vi "BK9120 Main Panel.vi"() -> ()   [LabVIEW 2014]
uses:
  BK9120/Serial_Config.ctl
  Meter_VI.ctl
  BK9120/B&K Precision 9120 series.lvclass
  <vilib>/Utility/error.llb/DialogType.ctl
panel:
  out "Const. Current":bool
  out "Const. Voltage":bool
  out "Enabled":bool
  in  "Output Enable":bool
  in  "Limit Setpoint":T1={"Voltage"=1.0, "Current"=1.0} caption="Measured" {"Current" min=0.0 max=1.2 step=0.001 scale=0.0..1.2 scale format="%#_5f"; "Voltage" min=0.0 max=73.0 step=0.1 scale=0.0..72.0 scale format="%#_5f"}
  out "Measured":T1 {"Current" min=0.0 max=1.2 step=0.001 scale=0.0..1.2 scale format="%#_5f"; "Voltage" min=0.0 max=73.0 step=0.1 scale=0.0..72.0 scale format="%#_5f"}
  in  "stop":bool
  out "Error Status":errorcluster
  in  "Connection":T3={"Serial Config"={"Baud"=38400, "Flow Ctl"=0, "Parity"=0}, "VISA resource name"="COM3", "Connect"=FALSE, "Status"="", "Connected"=FALSE} {"Serial Config"."Parity" items=["None", "Odd", "Even"]; "Serial Config"."Flow Ctl" items=["None"]; "Serial Config"."Baud" items=["4800"=4800, "9600"=9600, "19200"=19200, "38400"=38400]}
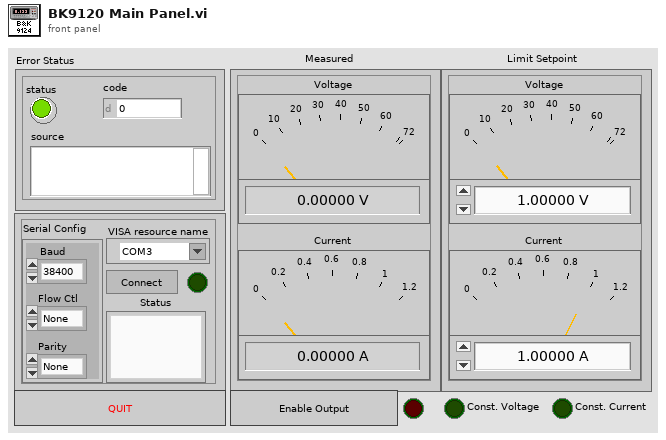
[diagram p1: front panel]
types:
  T1 = typedef "Meter_VI.ctl" = cluster{"Voltage":dbl, "Current":dbl}
  T2 = typedef "B&K Precision 9120 series.lvclass/Serial_Config.ctl" = cluster{"Baud":u32, "Flow Ctl":u16, "Parity":u16}
  T3 = cluster{"Serial Config":T2, "VISA resource name":refnum<visa-resource-name>, "Connect":bool, "Status":string, "Connected":bool}
  T4 = enum32{"invalid app kind", "Development System", "Run Time System", "Student Edition", "Embedded LabVIEW", "Evaluation", "Custom"}
  T5 = typedef "DialogType.ctl" = u16
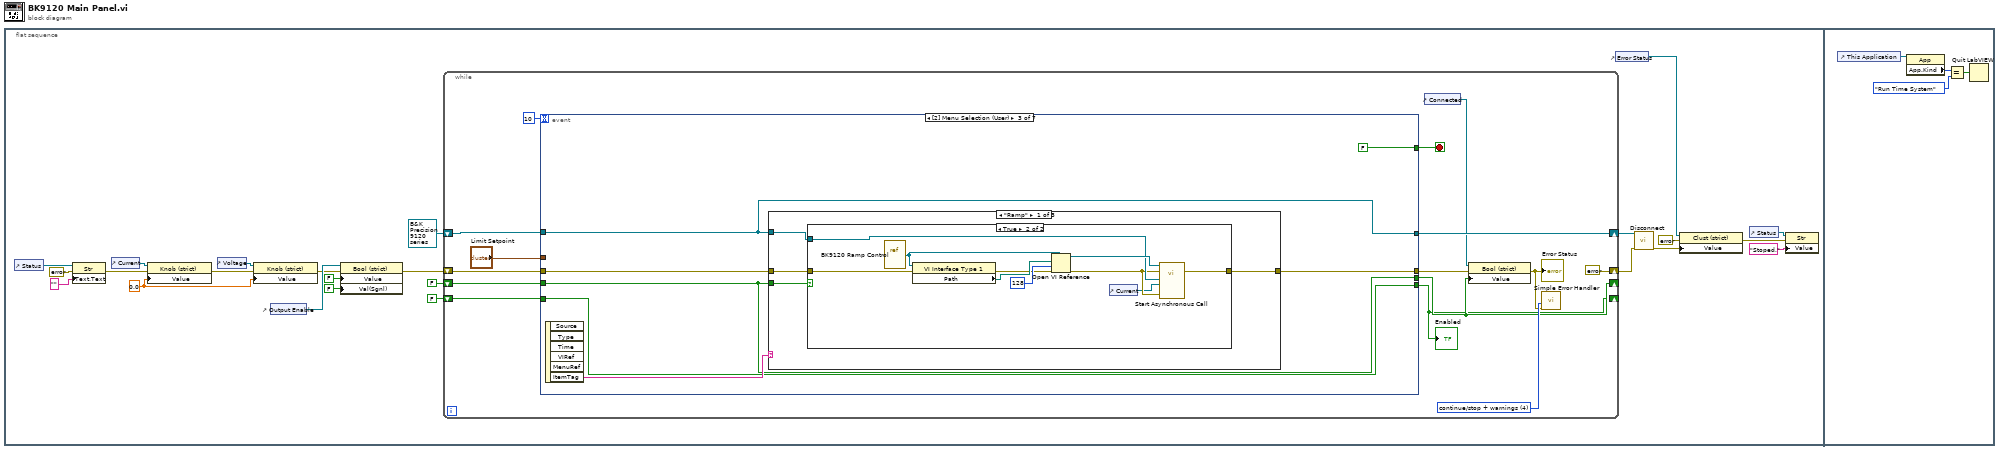
[diagram p0: block diagram]
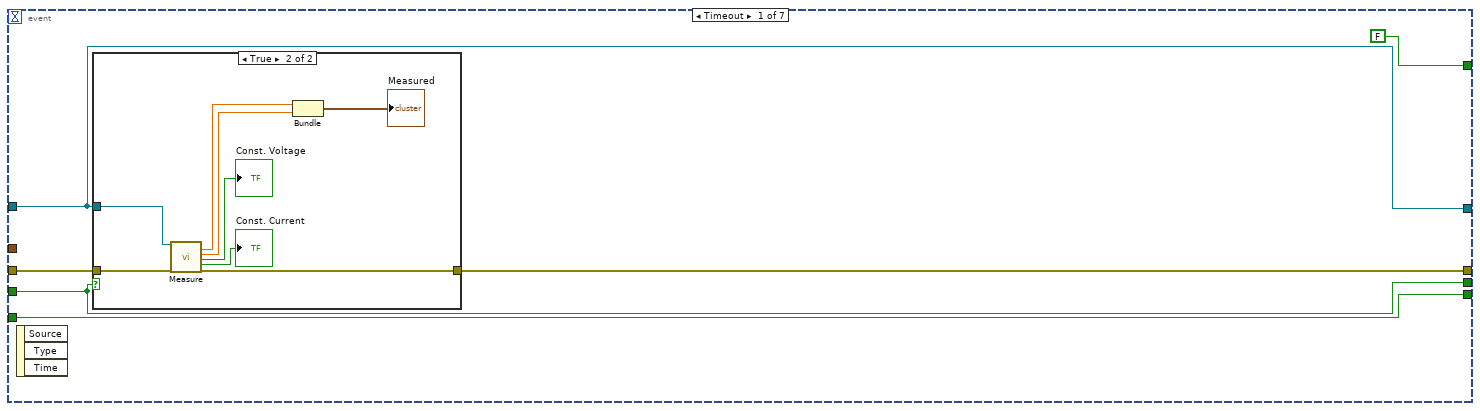
[diagram p2: hidden frame]
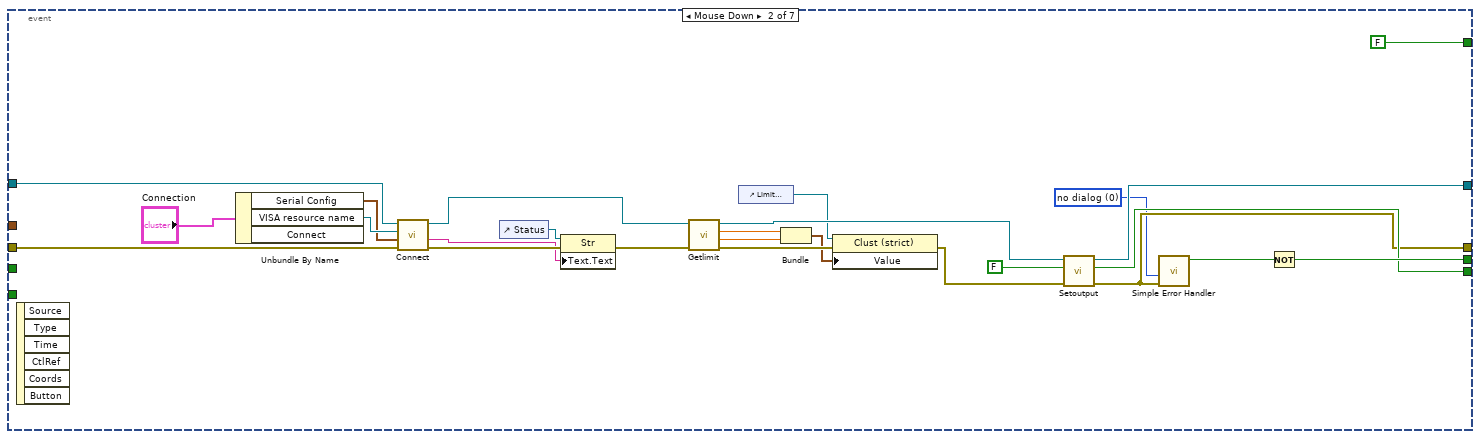
[diagram p4: hidden frame]
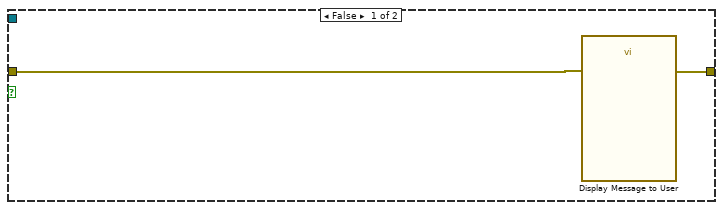
[diagram p5: hidden frame]
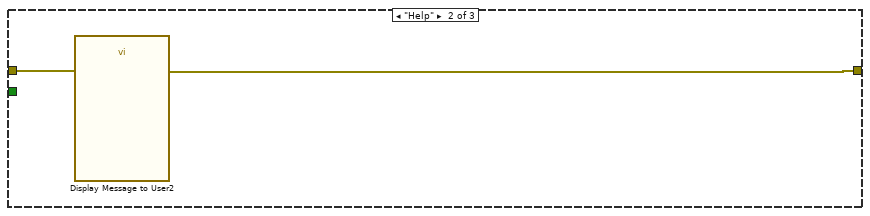
[diagram p6: hidden frame]
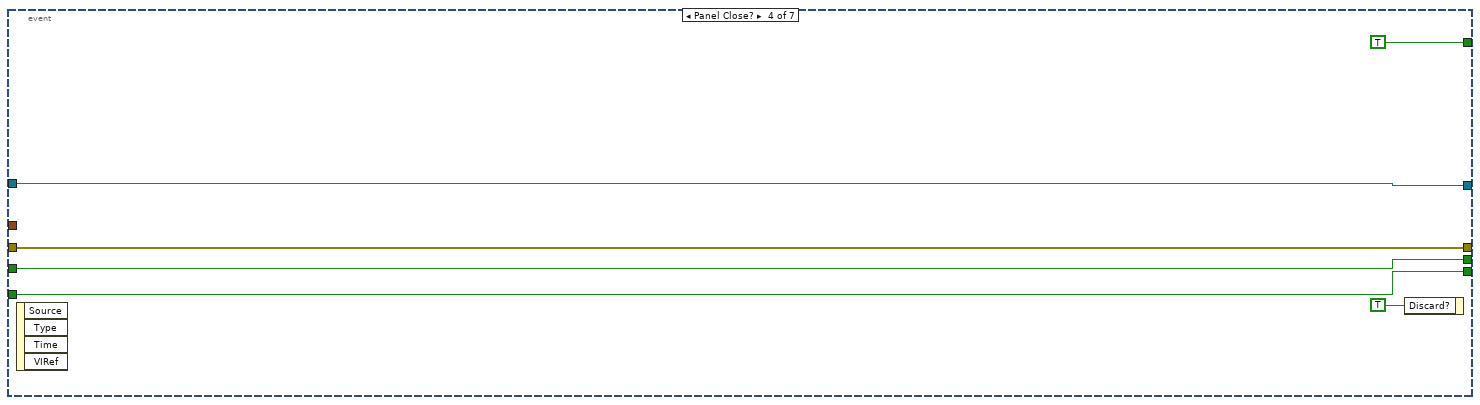
[diagram p8: hidden frame]
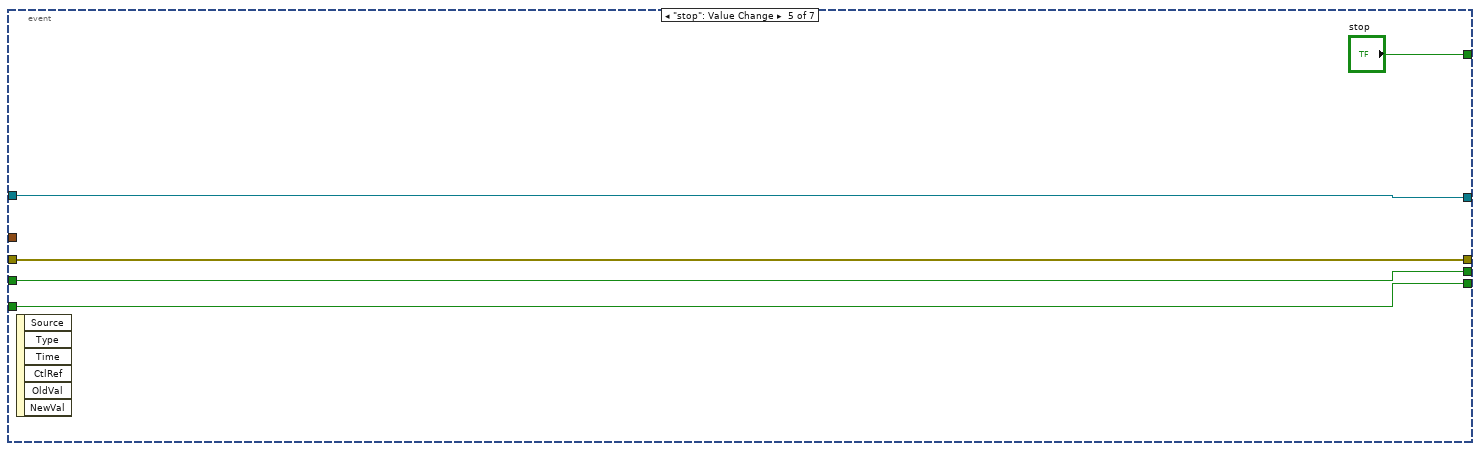
[diagram p9: hidden frame]
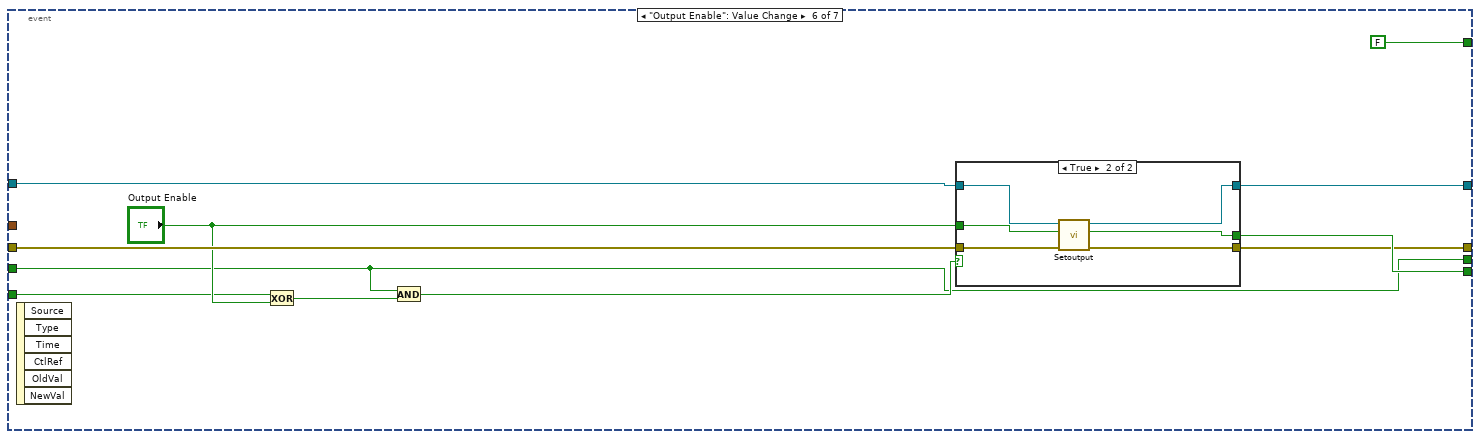
[diagram p10: hidden frame]
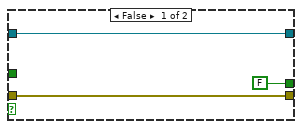
[diagram p11: hidden frame]
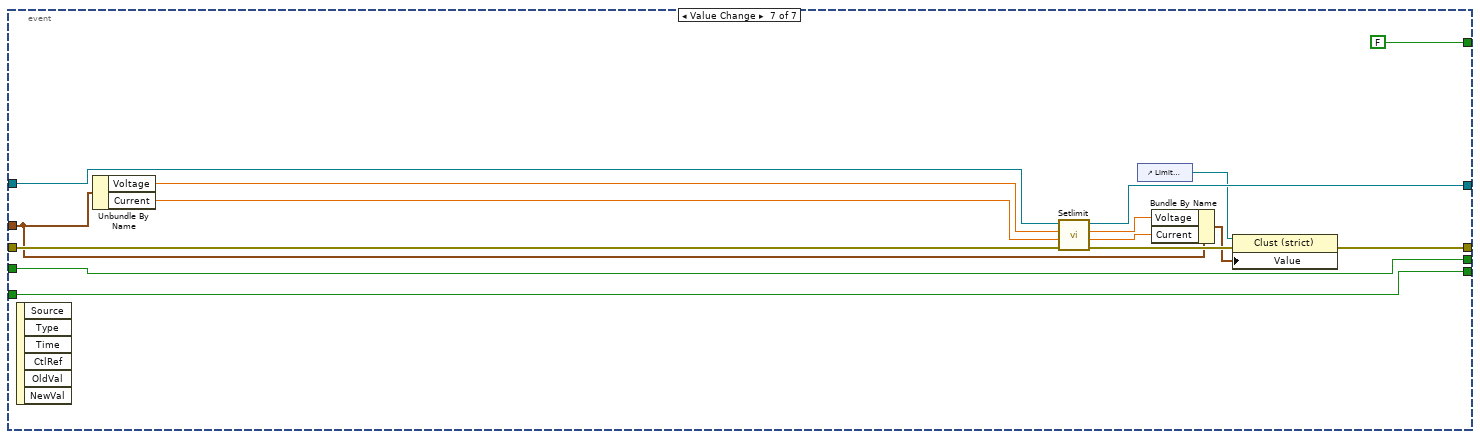
[diagram p12: hidden frame]
diagram:
  n1 = flat-sequence {
    frame #0 {
      w10 = 0.0 ("Value")
      n2 = control-ref of="Status"() -> (w18:refnum<vi>)
      n3 = property class="Str"(reference=w18, error in=errorcluster {"status"=FALSE, "code"=0, "source"=""} ("error in (no error)"), "Text.Text"="") -> (error out=w12:errorcluster)  [unwired: 1 out]
      n4 = control-ref of="Current"() -> (w13:refnum<vi>)
      n5 = property class="Knob (strict)"(reference=w13, error in=w12, "Value"=w10) -> (error out=w9:errorcluster)  [unwired: 1 out]
      n6 = control-ref of="Voltage"() -> (w11:refnum<vi>)
      n7 = property class="Knob (strict)"(reference=w11, error in=w9, "Value"=w10) -> (error out=w7:errorcluster)  [unwired: 1 out]
      n8 = control-ref of="Output Enable"() -> (w8:refnum<vi>)
      n9 = property class="Bool (strict)"(reference=w8, error in=w7, "Value"=FALSE ("Value (Signaling)"), "Val(Sgnl)"=FALSE ("Value (Signaling)")) -> (error out=w4:errorcluster)  [unwired: 1 out]
      n10 = while {
        shift-right: [errorcluster {"status"=FALSE, "code"=0, "source"=""} ("error out")] -> w22
        shift-left: w4 -> [w39]
        shift-right: [w38] -> w23
        shift-left: refnum<class "B&K Precision 9120 series.lvclass"> refnum ("B&K Precision 9120 series.lvclass") -> [w37]
        shift-right: [w30] -> _
        shift-left: FALSE -> [w33]
        shift-right: [w27] -> _
        shift-left: FALSE ("actual_state") -> [w29]
        stop <- w25 stop-if-true
        w35 = T5 4 items=["no dialog", "OK message", "continue or stop message", "OK message + warnings", "continue/stop + warnings"] ("type of dialog (OK msg:1)")
        n11 = event shown="[2] Menu Selection (User)" {
          selector: _ -> [_ _ _ _ _ _ _]
          dyn-events: _ -> [_ _ _ _ _ _ _]
          timeout: 10 -> [_ _ _ _ _ _ _]
          tunnel: w37 -> [w42 w79 w81 w111 w115 w127 w151]
          tunnel: w39 -> [w45 w76 w84 w110 w114 w124 w147]
          tunnel: [w44 w57 w83 w110 w114 w123 w141] -> w31
          tunnel: [w42 w61 w81 w111 w115 w125 w150] -> w38
          tunnel: w33 -> [w43 _ w80 w109 w113 w118 w140]
          tunnel: [w43 w71 w80 w109 w113 w118 w140] -> w30
          tunnel: [w41 w58 w85 w106 w112 w126 w139] -> w27
          tunnel: w29 -> [w41 _ w85 w106 w112 w121 w139]
          tunnel: "Limit Setpoint" -> [_ _ _ _ _ _ w138]
          tunnel: [FALSE ("stop") FALSE ("stop") FALSE ("stop") TRUE ("stop") "stop" FALSE ("stop") FALSE ("stop")] -> w25
          event Timeout {
            n12 = event-data() -> ()  [unwired: 1 in, 3 out]
            n13 = case shown="True" w43 {
              tunnel: w42 -> [_ w53]
              tunnel: w45 -> [w46 w52]
              tunnel: [w46 w49] -> w44
              frame False {
              }
              frame True {
                n14 = call "Measure.vi"("B&K Precision 9120 series in"=w53, "error in (no error)"=w52) -> ("Voltage"=w51:dbl, "Current"=w50:dbl, "CV"=→"Const. Voltage":bool, "CC"=→"Const. Current":bool, "error out"=w49:errorcluster)  [unwired: 12 in, 1 out]
                n15 = Bundle("Voltage"=w51, "Current"=w50) -> (→"Measured":cluster{"Voltage":dbl, "Current":dbl})  [unwired: 1 in]
              }
            }
          }
          event "Connection.Connect": Mouse Down {
            w56 = T5 0 items=["no dialog", "OK message", "continue or stop message", "OK message + warnings", "continue/stop + warnings"] ("type of dialog (OK msg:1)")
            n16 = event-data() -> ()  [unwired: 1 in, 6 out]
            n17 = Unbundle By Name("Connection") -> ("Serial Config"=w77:T2, "VISA resource name"=w78:refnum<visa-resource-name>)  [unwired: 1 out]
            n18 = call "Connect.vi"("error in (no error)"=w76, "Serial Config"=w77, "VISA resource name"=w78, "B&K Precision 9120 series in"=w79) -> ("error out"=w74:errorcluster, "result"=w73:string, "B&K Precision 9120 series out"=w69:refnum<class "B&K Precision 9120 series.lvclass">)  [unwired: 5 in]
            n19 = control-ref of="Status"() -> (w75:refnum<vi>)
            n20 = property class="Str"(reference=w75, error in=w74, "Text.Text"=w73) -> (error out=w67:errorcluster)  [unwired: 1 out]
            n21 = call "Getlimit.vi"("error in (no error)"=w67, "B&K Precision 9120 series in"=w69) -> ("error out"=w64:errorcluster, "Current read"=w65:dbl, "Voltage read"=w66:dbl, "B&K Precision 9120 series out"=w68:refnum<class "B&K Precision 9120 series.lvclass">)  [unwired: 6 in]
            n22 = control-ref of="Limit Setpoint"() -> (w63:refnum<vi>)
            n23 = Bundle("Voltage read"=w66, "Current read"=w65) -> (w62:cluster{"Voltage read":dbl, "Current read":dbl})  [unwired: 1 in]
            n24 = property class="Clust (strict)"(reference=w63, error in=w64, "Value"=w62) -> (error out=w60:errorcluster)  [unwired: 1 out]
            n25 = call "Setoutput.vi"("error in (no error)"=w60, "enable"=FALSE, "B&K Precision 9120 series in"=w68) -> ("error out"=w57:errorcluster, "actual_state"=w58:bool, "B&K Precision 9120 series out"=w61:refnum<class "B&K Precision 9120 series.lvclass">)  [unwired: 6 in]
            n26 = call <vilib>:"Simple Error Handler.vi"("type of dialog (OK msg:1)"=w56, "error in (no error)"=w57) -> ("error?"=w70:bool)  [unwired: 3 in, 4 out]
            n27 = Not(x=w70) -> (.not. x?=w71:bool)
          }
          event Menu Selection (User) {
            n28 = event-data() -> ("ItemTag"=w86:string)  [unwired: 1 in, 5 out]
            n29 = case shown="\"Ramp\"" w86 {
              tunnel: w84 -> [w90 w104 w105]
              tunnel: [w88 w103 w105] -> w83
              tunnel: w81 -> [w89 _ _]
              tunnel: w80 -> [w87 _ _]
              frame "Ramp" {
                n30 = case shown="True" w87 {
                  tunnel: w90 -> [w92 w98]
                  tunnel: w89 -> [_ w95]
                  tunnel: [w91 w96] -> w88
                  frame False {
                    n31 = call "Display Message to User"("error in (no error)"=w92) -> ("error out"=w91:errorcluster)  [unwired: 9 in, 1 out]
                  }
                  frame True {
                    n32 = vi-ref "BK9120 Ramp Control.vi"() -> (w100:refnum<vi>)
                    n33 = property class="VI Interface Type 1"(reference=w100, error in=w98) -> (error out=w97:errorcluster, "Path"=w99:path)  [unwired: 1 out]
                    n34 = Open VI Reference(type specifier VI Refnum (for type only)=w100, vi path=w99, options=128, error in (no error)=w97) -> (vi reference=w101:refnum<vi>, error out=w94:errorcluster)  [unwired: 2 in]
                    n35 = control-ref of="Current"() -> (w93:refnum<vi>)
                    n36 = call-by-ref "Start Asynchronous Call"(reference=w101, error in=w94, "Error In"=w94, "Current"=w93, "B&K In"=w95) -> (error out=w96:errorcluster)  [unwired: 7 in, 3 out]
                  }
                }
              }
              frame "Help" {
                n37 = call "Display Message to User2"("error in (no error)"=w104) -> ("error out"=w103:errorcluster)  [unwired: 9 in, 1 out]
              }
              frame Default {
              }
            }
          }
          event Panel Close? {
            n38 = event-data() -> ()  [unwired: 1 in, 4 out]
            n39 = event-data("Discard?"=TRUE) -> ()  [unwired: 1 in, 1 out]
          }
          event "stop": Value Change {
            n40 = event-data() -> ()  [unwired: 1 in, 6 out]
          }
          event "Output Enable": Value Change {
            n41 = event-data() -> ()  [unwired: 1 in, 6 out]
            n42 = Exclusive Or(1:"Output Enable", 2:w121) -> (0:w120:bool)
            n43 = And(x=w118, y=w120) -> (x .and. y?=w119:bool)
            n44 = case shown="True" w119 {
              tunnel: w127 -> [w130 w136]
              tunnel: [FALSE ("actual_state") w135] -> w126
              tunnel: [w130 w134] -> w125
              tunnel: w124 -> [w128 w133]
              tunnel: [w128 w132] -> w123
              tunnel: "Output Enable" -> [_ w131]
              frame False {
              }
              frame True {
                n45 = call "Setoutput.vi"("error in (no error)"=w133, "enable"=w131, "B&K Precision 9120 series in"=w136) -> ("error out"=w132:errorcluster, "actual_state"=w135:bool, "B&K Precision 9120 series out"=w134:refnum<class "B&K Precision 9120 series.lvclass">)  [unwired: 6 in]
              }
            }
          }
          event Value Change {
            n46 = event-data() -> ()  [unwired: 1 in, 6 out]
            n47 = Unbundle By Name(w138) -> ("Voltage"=w149:dbl, "Current"=w148:dbl)
            n48 = call "Setlimit.vi"("error in (no error)"=w147, "Current"=w148, "Voltage"=w149, "B&K Precision 9120 series in"=w151) -> ("error out"=w145:errorcluster, "Current read"=w143:dbl, "Voltage read"=w144:dbl, "B&K Precision 9120 series out"=w150:refnum<class "B&K Precision 9120 series.lvclass">)  [unwired: 4 in]
            n49 = control-ref of="Limit Setpoint"() -> (w146:refnum<vi>)
            n50 = Bundle By Name(cluster=w138, "Voltage"=w144, "Current"=w143) -> (w142:T1)
            n51 = property class="Clust (strict)"(reference=w146, error in=w145, "Value"=w142) -> (error out=w141:errorcluster)  [unwired: 1 out]
          }
        }
        "Enabled" <- w27
        n52 = control-ref of="Connected"() -> (w32:refnum<vi>)
        n53 = property class="Bool (strict)"(reference=w32, error in=w31, "Value"=w30) -> (error out=w28:errorcluster)  [unwired: 1 out]
        "Error Status" <- w28
        n54 = call <vilib>:"Simple Error Handler.vi"("type of dialog (OK msg:1)"=w35, "error in (no error)"=w28) -> ()  [unwired: 3 in, 5 out]
      }
      n55 = control-ref of="Error Status"() -> (w21:refnum<vi>)
      n56 = call "Disconnect.vi"("error in (no error)"=w22, "B&K Precision 9120 series in"=w23) -> ("error out"=w20:errorcluster)  [unwired: 9 in]
      n57 = property class="Clust (strict)"(reference=w21, error in=errorcluster {"status"=FALSE, "code"=0, "source"=""} ("error in (no error)"), "Value"=w20) -> (error out=w2:errorcluster)  [unwired: 1 out]
      n58 = control-ref of="Status"() -> (w3:refnum<vi>)
      n59 = property class="Str"(reference=w3, error in=w2, "Value"="Stoped.") -> ()  [unwired: 2 out]
    }
    frame #1 {
      n60 = control-ref of="This Application"() -> (w155:refnum<vi>)
      n61 = property class="App"(reference=w155) -> ("App.Kind"=w154:T4)  [unwired: 1 in, 2 out]
      n62 = Equal?(x=w154, y=T4."Run Time System") -> (x = y?=w152:bool)
      n63 = Quit LabVIEW(quit? (T)=w152) -> ()
    }
  }
